vi "Bursted Gate Test.vi"() -> ()   [LabVIEW 2015]
uses:
  Controls/Burst XCtl/Burst Data.ctl
  <vilib>/Analysis/NI_AALBase.lvlib
  Controls/Burst XCtl/Burst Control.xctl
panel:
  in  "T (s)":dbl=1.0
  out "Waveform Graph":dbl[](graph)
  in  "Burst":T1={"Active"=TRUE, "Delay (ms)"=0.0, "Duration (ms)"=100.0, "Ramp (ms)"=5.0, "Rate (Hz)"=5.0, "Trepeat (ms)"=0.0, "Repeat"=TRUE}
  in  "Sampling Rate (Hz)":dbl=50000.0
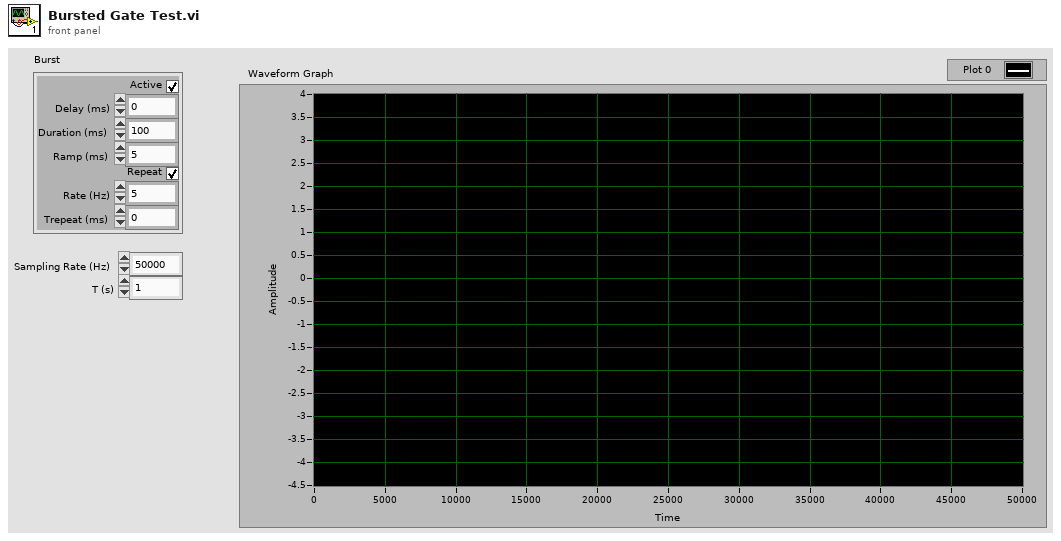
[diagram p1: front panel]
types:
  T1 = typedef "Burst Control.xctl/Burst Data.ctl" = cluster{"Active":bool, "Delay (ms)":dbl, "Duration (ms)":dbl, "Ramp (ms)":dbl, "Rate (Hz)":dbl, "Trepeat (ms)":dbl, "Repeat":bool}
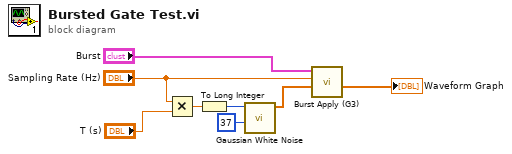
[diagram p0: block diagram]
diagram:
  n1 = Multiply(x="Sampling Rate (Hz)", y="T (s)") -> (x*y=w5:dbl)
  n2 = To Long Integer(number=w5) -> (32bit integer=w4:i32)
  n3 = call <vilib>:"Gaussian White Noise.vi"("seed"=37, "samples"=w4) -> ("Gaussian noise pattern"=w3:dbl[])  [unwired: 8 in, 1 out]
  n4 = call "Burst Apply (G3).vi"("Waveform in"=w3, "Sampling Rate (Hz)"="Sampling Rate (Hz)", "Burst"="Burst") -> ("Gated waveform"=→"Waveform Graph":dbl[])  [unwired: 7 in, 1 out]
